vi "Erase (array).vi"(8 "error in (no error)":errorcluster, 10 "Keys":string[](array[string]), 11 "Parameter to Hardware Map in":refnum<class "Parameter to Hardware Map.lvclass">) -> (0 "error out":errorcluster, 2 "Deleted Pairs":T1[](array[typedef]), 3 "Parameter to Hardware Map out":refnum<class "Parameter to Hardware Map.lvclass">)   [LabVIEW 2020, in "RxnRover.lvlib" / "Parameter to Hardware Map.lvclass"]
doc: "Removes all elements from the map specified in the array of keys."
uses:
  Parameter to Hardware Map.lvclass
  Pair.ctl
  Controller/Generic Plugin.lvclass
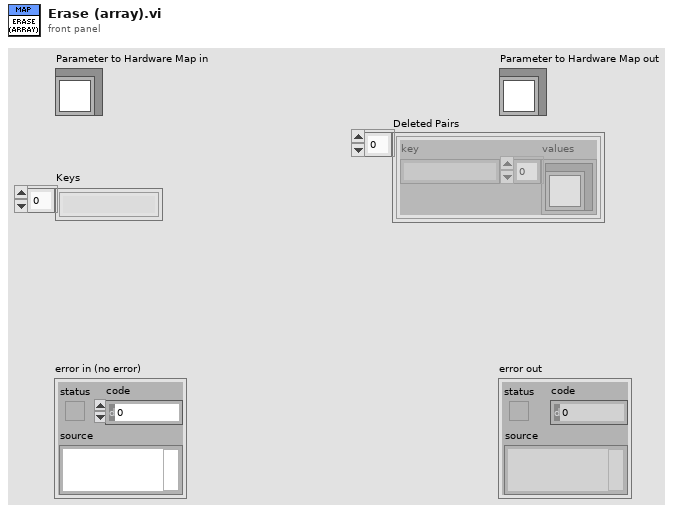
[diagram p1: front panel]
types:
  T1 = typedef "RxnRover.lvlib/Parameter to Hardware Map.lvclass/Pair.ctl" = cluster{"key":string, "values":refnum<class "Generic Plugin.lvclass">[]}
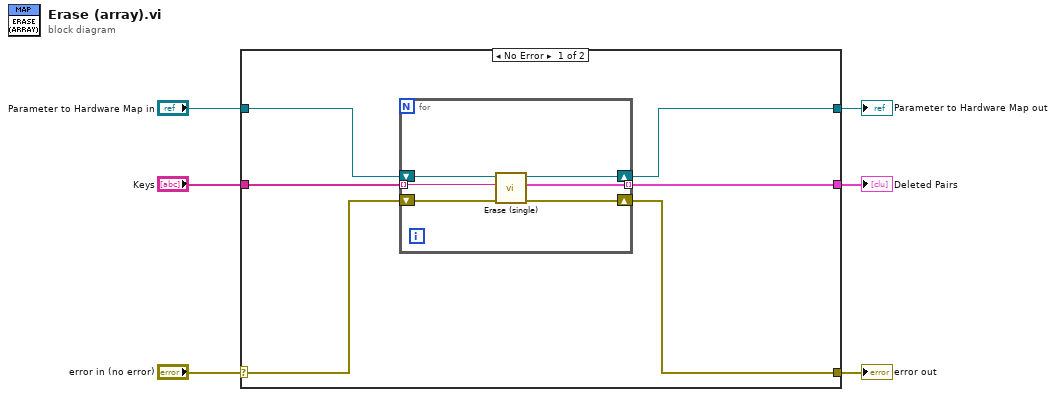
[diagram p0: block diagram]
diagram:
  n1 = case shown="No Error" "error in (no error)" {
    selector: "error in (no error)" -> [w10 w20]
    tunnel: [w8 w20] -> w5
    tunnel: [w9 w19] -> w3
    tunnel: "Parameter to Hardware Map in" -> [w12 w19]
    tunnel: "Keys" -> [w11 _]
    tunnel: [w7 _] -> w1
    frame No Error {
      n2 = for {
        tunnel: w11 -> [w16] mode=indexing
        shift-right: [w14] -> w9
        shift-left: w12 -> [w15]
        shift-right: [w17] -> w8
        shift-left: w10 -> [w18]
        tunnel: [w13] -> w7 mode=indexing
        n3 = call "Erase (single).vi"("error in (no error)"=w18, "Key"=w16, "Parameter to Hardware Map in"=w15) -> ("error out"=w17:errorcluster, "Deleted Pair"=w13:T1, "Parameter to Hardware Map out"=w14:refnum<class "Parameter to Hardware Map.lvclass">)  [unwired: 6 in]
      }
    }
    frame Error {
    }
  }
  "error out" <- w5
  "Parameter to Hardware Map out" <- w3
  "Deleted Pairs" <- w1
